vi "test_Export Instrument Addon Config.vi"(8 "error in (no error)":errorcluster, 11 "TestCase in":refnum<class "Instrument Addon Scripting API Custom Device Unit Tests.lvclass">) -> (0 "error out":errorcluster, 3 "TestCase out":refnum<class "Instrument Addon Scripting API Custom Device Unit Tests.lvclass">)   [LabVIEW 2021, in "Instrument Addon Scripting API Custom Device Unit Tests.lvclass"]
uses:
  Instrument Addon Scripting API Custom Device Unit Tests.lvclass
  Instrument Addon Scripting API Custom Device Unit Tests.lvclass/Instrument Addon Scripting API Custom Device Unit Tests.ctl
  <vilib>/addons/_JKI Toolkits/VI Tester/TestCase.llb/TestCase.lvclass
  APIs/Scripting API/Instrument Addon Scripting API.lvlib
  NationalInstruments.VeriStand.SystemDefinitionAPI
  <vilib>/NI VeriStand/Custom Device Tools/Custom Device Utility Library/Custom Device Utility Library.lvlib
  Addon/Addon Shared/SubVIs/Constants.vi
  Addon/Addon Shared/Instrument Addon Shared.lvlib
  <vilib>/NI VeriStand/Custom Device Tools/Custom Device Utility Library/NI VeriStand - Search for Item by GUID.vi
  C:/Program Files (x86)/National Instruments/LabVIEW 2020/vi.lib/addons/_JKI Toolkits/VI Tester/TestCase.llb/TestCase.lvclass
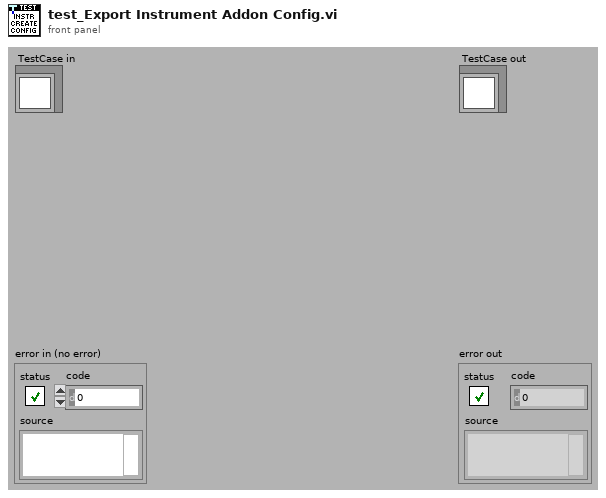
[diagram p1: front panel]
types:
  T1 = typedef "Custom Device API.lvlib/Custom Device Item Ref.ctl" = u64
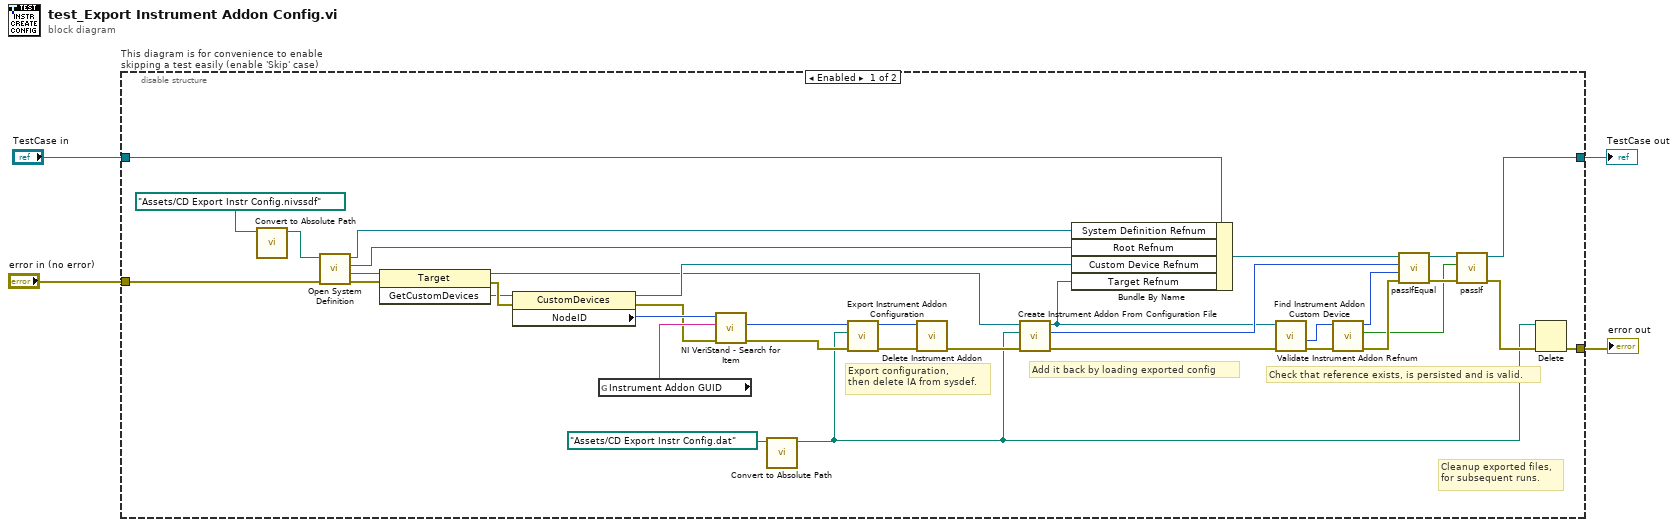
[diagram p0: block diagram]
diagram:
  n1 = disable-structure "This diagram is for convenience to enable skipping a test easily (enable 'Skip' case)" shown="Enabled" {
    disable-tunnel: "TestCase in" -> [w27 w44]
    disable-tunnel: [w12 w42] -> w1
    disable-tunnel: [w6 w43] -> w3
    disable-tunnel: "error in (no error)" -> [w40 w41]
    frame Enabled {
      # "Cleanup exported files,\nfor subsequent runs."
      # "Add it back by loading exported config"
      # "Export configuration,\nthen delete IA from sysdef."
      # "Check that reference exists, is persisted and is valid."
      n2 = call "Convert to Absolute Path.vi"("System Definition File"=path "Assets/CD Export Instr Config.nivssdf" ("SDF file")) -> ("Absolute Path"=w38:path)  [unwired: 10 in]
      n3 = call "Open System Definition.vi"("error in (no error)"=w40, "System Definition File"=w38) -> ("error out"=w34:errorcluster, "Target Refnum"=w33:refnum<k24>, "Root Refnum"=w25:refnum<k24>, "System Definition Refnum"=w26:refnum<k24>)  [unwired: 6 in]
      n4 = invoke class="Target" method="GetCustomDevices"(reference=w33, error in=w34) -> (reference out=w23:refnum<k24>, error out=w36:errorcluster, "GetCustomDevices"=w35:refnum<k24>)  [unwired: 1 in]
      n5 = property class="CustomDevices"(reference=w35, error in=w36) -> (reference out=w24:refnum<k24>, error out=w30:errorcluster, "NodeID"=w32:u64)
      n6 = global read "Constants.vi" "Instrument Addon GUID"() -> (w31:string)
      n7 = call-poly <vilib>:"NI VeriStand - Search for Item.vi"("error in"=w30, "Item GUID"=w31, "Section Ref in"=w32) -> ("error out"=w29:errorcluster, "Item Ref"=w28:T1)  [unwired: 5 in, 2 out]
      n8 = call "Convert to Absolute Path.vi"("System Definition File"=path "Assets/CD Export Instr Config.dat" ("SDF file")) -> ("Absolute Path"=w5:path)  [unwired: 10 in]
      n9 = call "Export Instrument Addon Configuration.vi"("error in (no error)"=w29, "export file path"=w5, "instrument addon refnum in"=w28) -> ("error out"=w9:errorcluster, "instrument addon refnum out"=w10:T1)  [unwired: 7 in]
      n10 = call "Delete Instrument Addon.vi"("error in (no error)"=w9, "instrument addon refnum"=w10) -> ("error out"=w8:errorcluster)  [unwired: 9 in]
      n11 = call "Create Instrument Addon From Configuration File.vi"("error in (no error)"=w8, "configuration file path"=w5, "target in"=w23) -> ("error out"=w15:errorcluster, "instrument addon refnum"=w13:T1, "target out"=w11:refnum<k24>)  [unwired: 6 in]
      n12 = Bundle By Name(cluster=w27, "System Definition Refnum"=w26, "Root Refnum"=w25, "Custom Device Refnum"=w24, "Target Refnum"=w11) -> (w14:refnum<class "Instrument Addon Scripting API Custom Device Unit Tests.lvclass">)
      n13 = call "Find Instrument Addon Custom Device.vi"("error in"=w15, "target in"=w11) -> ("error out"=w21:errorcluster, "NodeID"=w22:u64)  [unwired: 7 in, 1 out]
      n14 = call "Validate Instrument Addon Refnum.vi"("Error In"=w21, "Refnum In"=w22) -> ("Error Out"=w20:errorcluster, "Is Instrument Addon?"=w16:bool, "Refnum Out"=w19:T1)  [unwired: 7 in]
      n15 = call-dynamic "passIfEqual.vi"("error in (no error)"=w20, "y"=w19, "x"=w13, "TestCase in"=w14) -> ("error out"=w18:errorcluster, "TestCase out"=w17:refnum<class "Instrument Addon Scripting API Custom Device Unit Tests.lvclass">)  [unwired: 6 in]
      n16 = call-dynamic "passIf.vi"("error in (no error)"=w18, "pass"=w16, "TestCase in"=w17) -> ("error out"=w7:errorcluster, "TestCase out"=w12:refnum<class "Instrument Addon Scripting API Custom Device Unit Tests.lvclass">)  [unwired: 7 in]
      n17 = Delete(path (use dialog)=w5, error in=w7) -> (error out=w6:errorcluster)  [unwired: 3 in, 2 out]
    }
    frame Disabled {
      # "skip test result while test is under development"
      n18 = call <vilib>:"skip.vi"("error in (no error)"=w41, "TestCase in"=w44) -> ("error out"=w43:errorcluster, "TestCase out"=w42:refnum<class "Instrument Addon Scripting API Custom Device Unit Tests.lvclass">)  [unwired: 8 in]
    }
  }
  "error out" <- w3
  "TestCase out" <- w1
